vi "Delete Data Folder.vi"(5 "Files Generated by Build":path[](array[path]), 6 "Top Level/Always Included VIs":path[](array[path]), 7 "Destination Path":path, 8 "error in (no error)":errorcluster, 9 "Target Name":string, 10 "Build Specification Name":string, 11 "Project Path":path) -> (0 "error out":errorcluster)   [LabVIEW 2019, in "Build VIs.lvlib"]
uses:
  Build VIs.lvlib
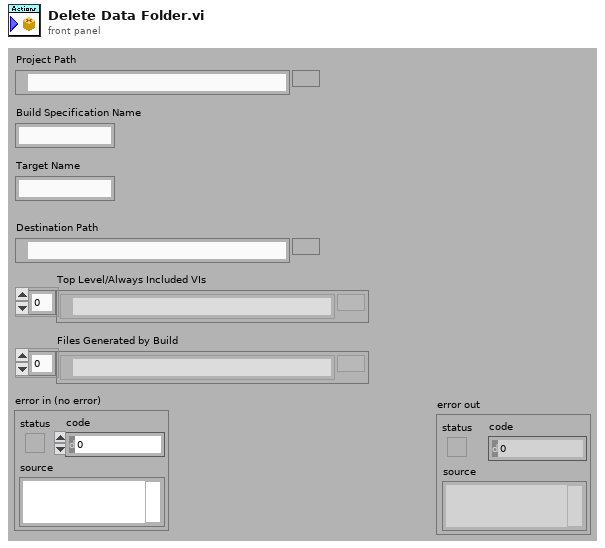
[diagram p1: front panel]
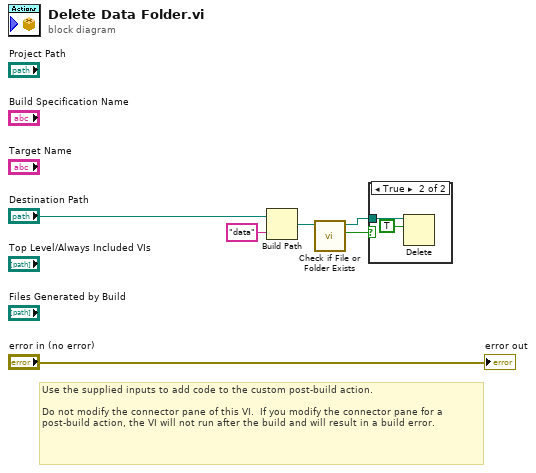
[diagram p0: block diagram]
diagram:
  # "Use the supplied inputs to add code to the custom post-build action.\n\nDo not modify the connector pane of this VI.  If you modify the connector pane for a post-build action, the VI will not run after the build and will result in a build error."
  n1 = Build Path(base path="Destination Path", name or relative path="data") -> (appended path=w3:path)
  n2 = call <vilib>:"Check if File or Folder Exists.vi"("path"=w3) -> ("file or folder exists?"=w2:bool, "dup path"=w1:path)  [unwired: 8 in, 1 out]
  n3 = case shown="True" w2 {
    tunnel: w1 -> [_ w8]
    frame False {
    }
    frame True {
      n4 = Delete(path (use dialog)=w8, entire hierarchy (F)=TRUE) -> ()  [unwired: 3 in, 3 out]
    }
  }
  "error out" <- "error in (no error)"
